vi "Create Default Attributes.vi"(5 "Unique ID":string, 7 "Process Executive Ref":refnum<data-value>, 11 "Stop Spot Free Rinse in":refnum<class "Stop Spot Free Rinse.lvclass">) -> (3 "Stop Spot Free Rinse out":refnum<class "Stop Spot Free Rinse.lvclass">)   [LabVIEW 2019, in "Stop Spot Free Rinse.lvclass"]
uses:
  <vilib>/gpm_packages/@cs/Car-wash/Source/Process Steps/Stop Spot Free Rinse/Stop Spot Free Rinse.lvclass
  <vilib>/gpm_packages/@cs/test-executive/Source/Test Executive/ITestExecutive/ITest Executive.lvclass
  91ab7ded-5a84-47c7-8c0f-290c3a085cfb.vi
  <vilib>/Utility/error.llb/Error Cluster From Error Code.vi
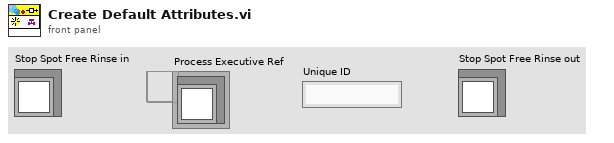
[diagram p1: front panel]
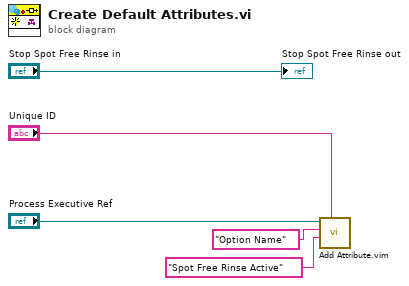
[diagram p0: block diagram]
diagram:
  n1 = call "Add Attribute.vim"("ID"="Unique ID", "Attribute"="Spot Free Rinse Active" ("Item Name"), "Attribute Name"="Option Name" ("Item Name"), "Test Executive Ref"="Process Executive Ref") -> ()  [unwired: 4 in, 4 out]
  "Stop Spot Free Rinse out" <- "Stop Spot Free Rinse in"
